vi "Resize.Align Ctrl with Ctrl.vi"(4 "Move Ctrl Ref Location":T1(ring), 5 "dY":i32, 6 "Ref Ctrl Corner":T2(ring), 7 "dX":i32, 8 "error in":errorcluster, 10 "Move Ctrl":refnum<vi>, 11 "Ref Ctrl":refnum<vi>) -> (0 "error out":errorcluster, 2 "Move Ctrl Out":refnum<vi>, 3 "Ref Ctrl Out":refnum<vi>)   [LabVIEW 2024, in "EQMF.lvlib" / "Controls.lvlib"]
doc: "This VI aligns two controls. The referenced corner of the second control is moved to within Dx and Dy distance (in pixels) from the referenced corner of the first control.\n\nINPUTS:\n<B>dX</B> - The delta X position.\n<B>dY</B> - The delta Y position.\n<B>Ref Ctrl</B> - Control reference that stays stationary.\n<B>Move Ctrl</B> - Control reference that is moved.\n<B>Rel Ctrl Corner</B> - An enumerator specifying the corner that is to be aligned.\n<B>Move Ctrl Ref Location</B> - An enumerator specifying the corner that is to be aligned.\n\nOUTPUTS:\n<B>Ref Ctrl</B> - Duplicate control reference that stays stationary.\n<B>Move Ctrl</B> - Duplicate control reference that is moved.\n\nERRORS: \nAn error will be generated if one of the controls are the incorrect type or if the control reference is invalid."
uses:
  Controls.lvlib
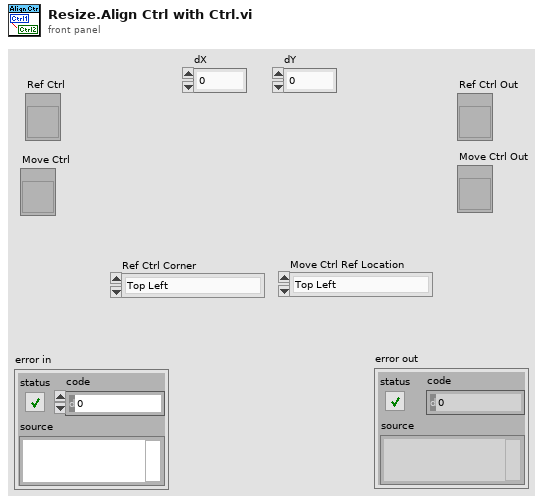
[diagram p1: front panel]
types:
  T1 = enum16{"Top Left", "Top Right", "Bottom Left", "Bottom Right", "Left", "Right", "Top", "Bottom"}
  T2 = enum16{"Top Left", "Top Right", "Bottom Left", "Bottom Right"}
  T3 = typedef "EQMF.lvlib/Controls.lvlib/Resize, Object Position Info.ctl" = cluster{"Left":i32, "Right":i32, "Width":i32, "Top":i32, "Bottom":i32, "Height":i32}
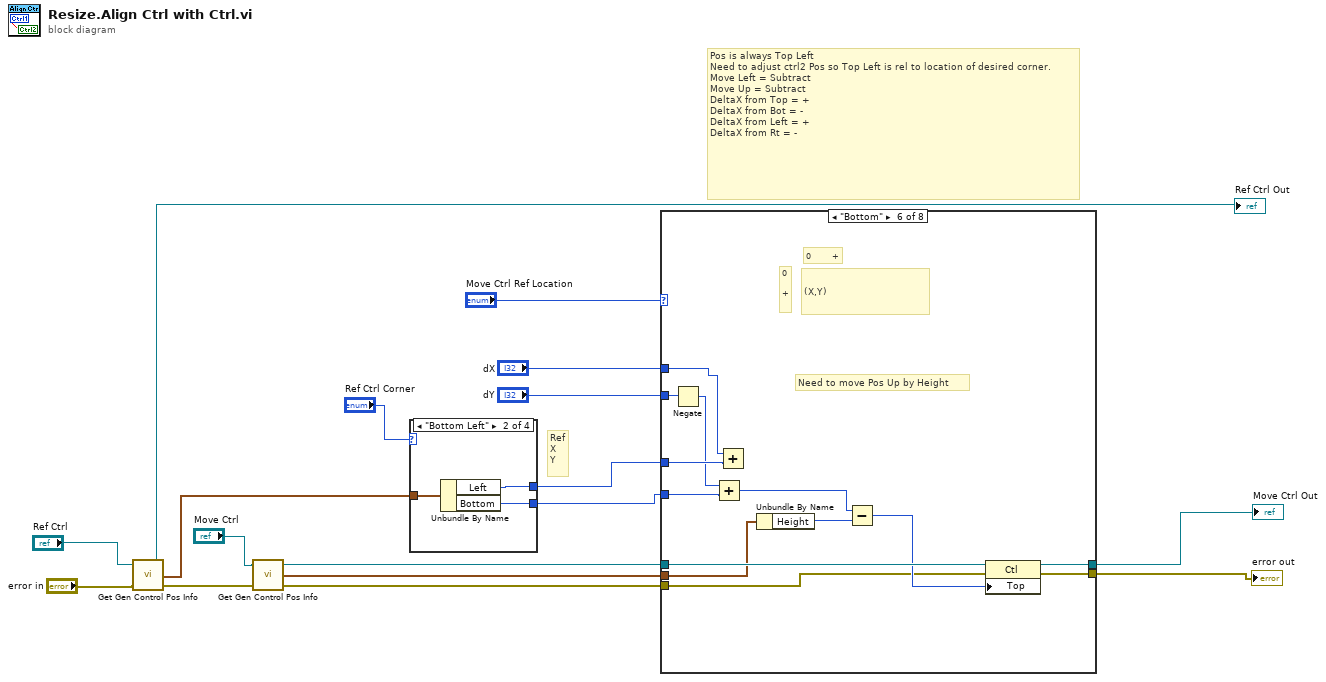
[diagram p0: block diagram]
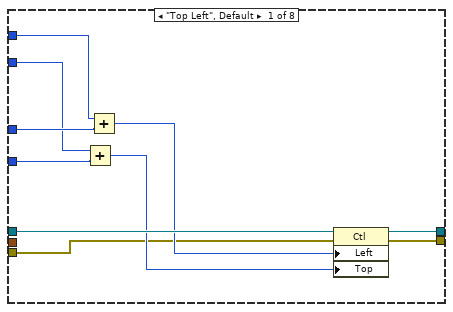
[diagram p2: hidden frame]
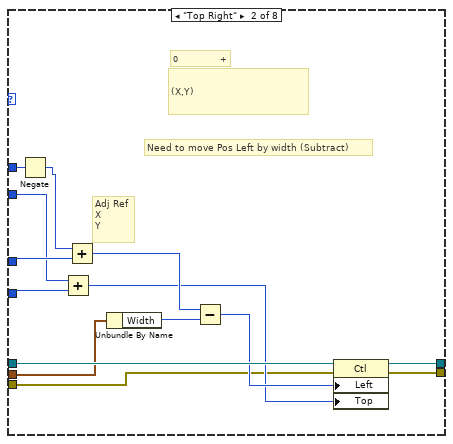
[diagram p3: hidden frame]
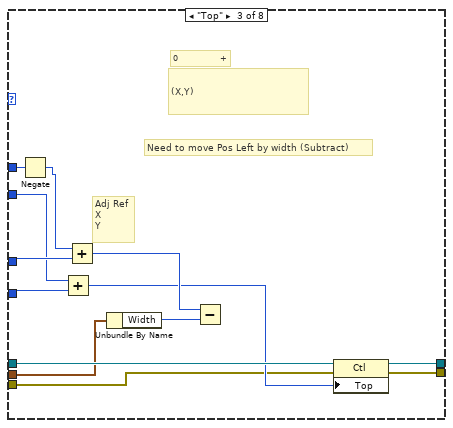
[diagram p4: hidden frame]
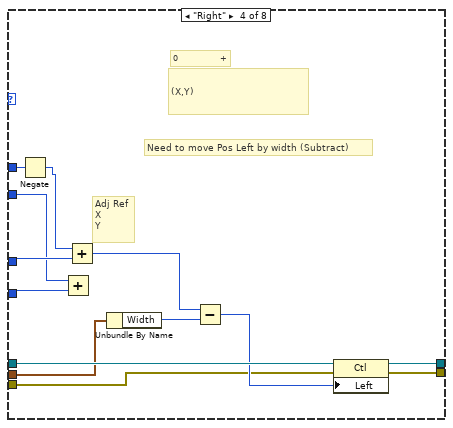
[diagram p5: hidden frame]
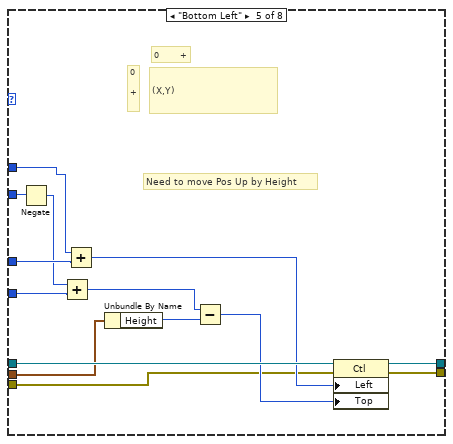
[diagram p6: hidden frame]
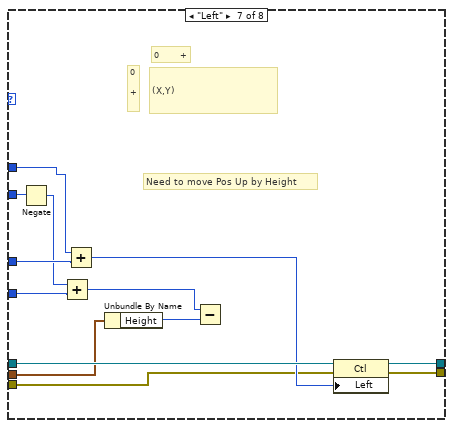
[diagram p7: hidden frame]
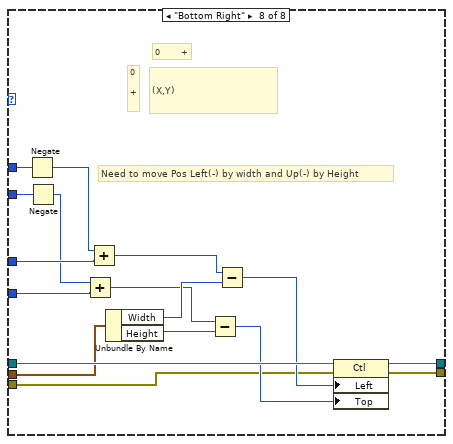
[diagram p8: hidden frame]
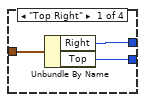
[diagram p9: hidden frame]
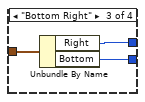
[diagram p10: hidden frame]
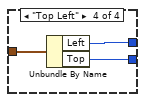
[diagram p11: hidden frame]
diagram:
  # "Pos is always Top Left\nNeed to adjust ctrl2 Pos so Top Left is rel to location of desired corner.\nMove Left = Subtract\nMove Up = Subtract\nDeltaX from Top = +\nDeltaX from Bot = -\nDeltaX from Left = +\nDeltaX from Rt = -"
  # "Ref\nX\nY"
  n1 = call "Get Gen Control Pos Info.vi"("error in"="error in", "Ctl Refnum"="Ref Ctrl") -> ("error out"=w5:errorcluster, "Pos Info"=w6:T3, "Ctl Refnum Out"=→"Ref Ctrl Out":refnum<vi>)  [unwired: 1 in]
  n2 = call "Get Gen Control Pos Info.vi"("error in"=w5, "Ctl Refnum"="Move Ctrl") -> ("error out"=w7:errorcluster, "Pos Info"=w15:T3, "Ctl Refnum Out"=w14:refnum<vi>)  [unwired: 1 in]
  n3 = case shown="\"Bottom Left\"" "Ref Ctrl Corner" {
    tunnel: w6 -> [w20 w23 w26 w29]
    tunnel: [w19 w22 w25 w28] -> w12
    tunnel: [w18 w21 w24 w27] -> w13
    frame "Top Right" {
      n4 = Unbundle By Name(w20) -> ("Right"=w19:i32, "Top"=w18:i32)
    }
    frame "Bottom Left" {
      n5 = Unbundle By Name(w23) -> ("Left"=w22:i32, "Bottom"=w21:i32)
    }
    frame "Bottom Right" {
      n6 = Unbundle By Name(w26) -> ("Right"=w25:i32, "Bottom"=w24:i32)
    }
    frame "Top Left" {
      n7 = Unbundle By Name(w29) -> ("Left"=w28:i32, "Top"=w27:i32)
    }
  }
  n8 = case shown="\"Bottom\"" "Move Ctrl Ref Location" {
    tunnel: w15 -> [_ w50 w63 w76 w90 w103 w116 w133]
    tunnel: w12 -> [w36 w46 w60 w72 w84 w97 w111 w127]
    tunnel: w13 -> [w35 w47 w61 w73 w86 w99 w113 w128]
    tunnel: w14 -> [w39 w53 w66 w79 w93 w106 w119 w136]
    tunnel: [w38 w52 w65 w78 w92 w105 w118 w135] -> w2
    tunnel: [w37 w51 w64 w77 w91 w104 w117 w134] -> w8
    tunnel: "dY" -> [w33 w45 w59 w71 w82 w96 w109 w122]
    tunnel: "dX" -> [w34 w42 w56 w69 w87 w100 w114 w124]
    tunnel: w7 -> [w30 w40 w54 w67 w80 w94 w107 w120]
    frame "Top Left", Default {
      n9 = Add(x=w33, y=w35) -> (x+y=w31:i32)
      n10 = Add(x=w34, y=w36) -> (x+y=w32:i32)
      n11 = property class="Ctl"(reference=w39, error in=w30, "Left"=w32, "Top"=w31) -> (reference out=w38:refnum<vi>, error out=w37:errorcluster)
    }
    frame "Top Right" {
      # "Adj Ref\nX\nY"
      # "0              +"
      # "Need to move Pos Left by width (Subtract)"
      # "(X,Y)"
      n12 = Negate(x=w42) -> (-x=w41:i32)
      n13 = Add(x=w45, y=w47) -> (x+y=w43:i32)
      n14 = Add(x=w41, y=w46) -> (x+y=w44:i32)
      n15 = Unbundle By Name(w50) -> ("Width"=w49:i32)
      n16 = Subtract(x=w44, y=w49) -> (x-y=w48:i32)
      n17 = property class="Ctl"(reference=w53, error in=w40, "Left"=w48, "Top"=w43) -> (reference out=w52:refnum<vi>, error out=w51:errorcluster)
    }
    frame "Top" {
      # "Adj Ref\nX\nY"
      # "0              +"
      # "Need to move Pos Left by width (Subtract)"
      # "(X,Y)"
      n18 = Negate(x=w56) -> (-x=w55:i32)
      n19 = Add(x=w59, y=w61) -> (x+y=w57:i32)
      n20 = Add(x=w55, y=w60) -> (x+y=w58:i32)
      n21 = Unbundle By Name(w63) -> ("Width"=w62:i32)
      n22 = Subtract(x=w58, y=w62) -> ()  [unwired: 1 out]
      n23 = property class="Ctl"(reference=w66, error in=w54, "Top"=w57) -> (reference out=w65:refnum<vi>, error out=w64:errorcluster)
    }
    frame "Right" {
      # "Adj Ref\nX\nY"
      # "0              +"
      # "Need to move Pos Left by width (Subtract)"
      # "(X,Y)"
      n24 = Negate(x=w69) -> (-x=w68:i32)
      n25 = Add(x=w71, y=w73) -> ()  [unwired: 1 out]
      n26 = Add(x=w68, y=w72) -> (x+y=w70:i32)
      n27 = Unbundle By Name(w76) -> ("Width"=w75:i32)
      n28 = Subtract(x=w70, y=w75) -> (x-y=w74:i32)
      n29 = property class="Ctl"(reference=w79, error in=w67, "Left"=w74) -> (reference out=w78:refnum<vi>, error out=w77:errorcluster)
    }
    frame "Bottom Left" {
      # "0       +"
      # "0\n\n+"
      # "Need to move Pos Up by Height"
      # "(X,Y)"
      n30 = Negate(x=w82) -> (-x=w81:i32)
      n31 = Add(x=w81, y=w86) -> (x+y=w85:i32)
      n32 = Add(x=w87, y=w84) -> (x+y=w83:i32)
      n33 = Unbundle By Name(w90) -> ("Height"=w89:i32)
      n34 = Subtract(x=w85, y=w89) -> (x-y=w88:i32)
      n35 = property class="Ctl"(reference=w93, error in=w80, "Left"=w83, "Top"=w88) -> (reference out=w92:refnum<vi>, error out=w91:errorcluster)
    }
    frame "Bottom" {
      # "0       +"
      # "0\n\n+"
      # "Need to move Pos Up by Height"
      # "(X,Y)"
      n36 = Negate(x=w96) -> (-x=w95:i32)
      n37 = Add(x=w95, y=w99) -> (x+y=w98:i32)
      n38 = Add(x=w100, y=w97) -> ()  [unwired: 1 out]
      n39 = Unbundle By Name(w103) -> ("Height"=w102:i32)
      n40 = Subtract(x=w98, y=w102) -> (x-y=w101:i32)
      n41 = property class="Ctl"(reference=w106, error in=w94, "Top"=w101) -> (reference out=w105:refnum<vi>, error out=w104:errorcluster)
    }
    frame "Left" {
      # "0       +"
      # "0\n\n+"
      # "Need to move Pos Up by Height"
      # "(X,Y)"
      n42 = Negate(x=w109) -> (-x=w108:i32)
      n43 = Add(x=w108, y=w113) -> (x+y=w112:i32)
      n44 = Add(x=w114, y=w111) -> (x+y=w110:i32)
      n45 = Unbundle By Name(w116) -> ("Height"=w115:i32)
      n46 = Subtract(x=w112, y=w115) -> ()  [unwired: 1 out]
      n47 = property class="Ctl"(reference=w119, error in=w107, "Left"=w110) -> (reference out=w118:refnum<vi>, error out=w117:errorcluster)
    }
    frame "Bottom Right" {
      # "0       +"
      # "0\n\n+"
      # "Need to move Pos Left(-) by width and Up(-) by Height"
      # "(X,Y)"
      n48 = Negate(x=w124) -> (-x=w123:i32)
      n49 = Negate(x=w122) -> (-x=w121:i32)
      n50 = Add(x=w121, y=w128) -> (x+y=w126:i32)
      n51 = Add(x=w123, y=w127) -> (x+y=w125:i32)
      n52 = Unbundle By Name(w133) -> ("Width"=w130:i32, "Height"=w132:i32)
      n53 = Subtract(x=w126, y=w132) -> (x-y=w131:i32)
      n54 = Subtract(x=w125, y=w130) -> (x-y=w129:i32)
      n55 = property class="Ctl"(reference=w136, error in=w120, "Left"=w129, "Top"=w131) -> (reference out=w135:refnum<vi>, error out=w134:errorcluster)
    }
  }
  "error out" <- w8
  "Move Ctrl Out" <- w2
